vi "DP I-O Append Data.vi"(0 "DataAcq":T1, 5 "Waveform":dbl[](array[numeric]), 9 "Processed data":dbl[](array[numeric]), 11 "error in (no error)":errorcluster) -> (15 "error out":errorcluster)   [LabVIEW 2020]
uses:
  Typedefs/DP-DataAcq.ctl
  <vilib>/Utility/file.llb/Write To Spreadsheet File (DBL).vi
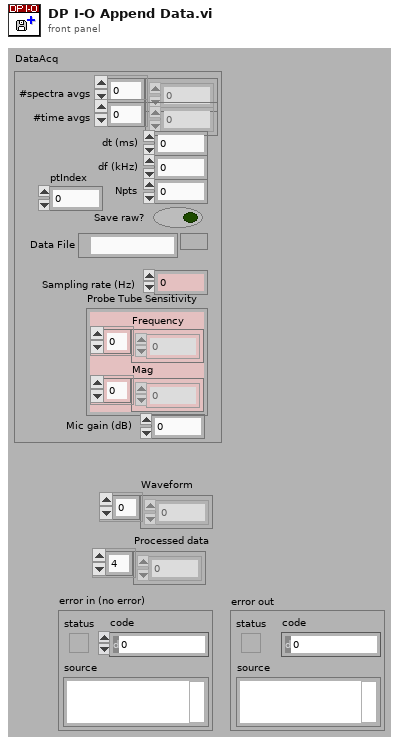
[diagram p1: front panel]
types:
  T1 = typedef "DP-DataAcq.ctl" = cluster{"#spectra avgs":i32[], "#time avgs":i32[], "dt (ms)":dbl, "df (kHz)":dbl, "Npts":i32, "Save raw?":bool, "Data File":path, "Sampling rate (Hz)":dbl, "Probe Tube Sensitivity":cluster{"Frequency":dbl[], "Mag":dbl[]}, "Mic gain (dB)":dbl, "ptIndex":i32}
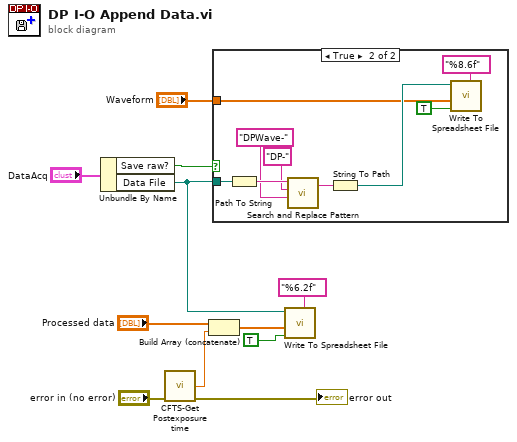
[diagram p0: block diagram]
diagram:
  n1 = Unbundle By Name("DataAcq") -> ("Save raw?"=w2:bool, "Data File"=w1:path)
  n2 = call "CFTS-Get Postexposure time.vi"("error in (no error)"="error in (no error)") -> ("Postexposure Time (min)"=w5:dbl, "error out"=→"error out":errorcluster)  [unwired: 13 in]
  n3 = Build Array (concatenate)("Processed data", w5) -> (w6:dbl[])
  n4 = case shown="True" w2 {
    tunnel: w1 -> [_ w16]
    tunnel: "Waveform" -> [_ w14]
    frame False {
    }
    frame True {
      n5 = Path To String(path=w16) -> (string=w20:string)
      n6 = call <vilib>:"Search and Replace Pattern.vi"("string"=w20, "regular expression (\"\")"="DP-" ("regular expression (\"\")"), "replace string (\"\")"="DPWave-" ("regular expression (\"\")")) -> ("result string"=w17:string)  [unwired: 2 in, 1 out]
      n7 = String To Path(string=w17) -> (path=w15:path)
      n8 = call-poly <vilib>:"Write To Spreadsheet File.vi"("format (%.3f)"="%8.6f", "append to file? (new file:F)"=TRUE, "1D data"=w14, "file path (dialog if empty)"=w15) -> ()  [unwired: 4 in, 1 out]
    }
  }
  n9 = call-poly <vilib>:"Write To Spreadsheet File.vi"("format (%.3f)"="%6.2f", "append to file? (new file:F)"=TRUE, "1D data"=w6, "file path (dialog if empty)"=w1) -> ()  [unwired: 4 in, 1 out]
